vi "LC1_MS_Main.vi"() -> ()   [LabVIEW 2016, in "DNP3_Master_Station_Template.lvlib"]
uses:
  DNP3_Master_Station_Template.lvlib
  Program Files (x86)/National Instruments/LabVIEW 2016/examples/DNP3/Get Started/Master/SubVI/Tab_Master.ctl
  <vilib>/DNP3/DNP3_Master/Response Type.ctl
  <vilib>/Utility/error.llb/DialogType.ctl
  Global_An_In_Var.vi
  Global_An_Out_Mode.vi
  Global_An_Out_Var.vi
  <vilib>/DNP3/DNP3_Master/Send Poll Analog Input By AllPoints (Blocking).vi
  <vilib>/DNP3/DNP3_Master/Read Analog Input.vi
  <vilib>/DNP3/DNP3_Master/Send Analog Output Block (Blocking).vi
  Global_Bin_In_Var.vi
  Global_Bin_Out_Mode.vi
  <vilib>/DNP3/DNP3_Master/Send Poll Binary Input By AllPoints (Blocking).vi
  <vilib>/DNP3/DNP3_Master/Read Binary Input.vi
  <vilib>/DNP3/DNP3_Master/Send CROB (Blocking).vi
  <vilib>/DNP3/DNP3_Master.lvlib
  <resource>/objmgr/dnp3.rc
panel:
  out "object flags":u8[](array[numeric]) format="%08b"
  in  "Channel Setting":T1
  in  "serial port":u16=1
  in  "baud rate (9600)":u32=9600
  in  "Stop":bool
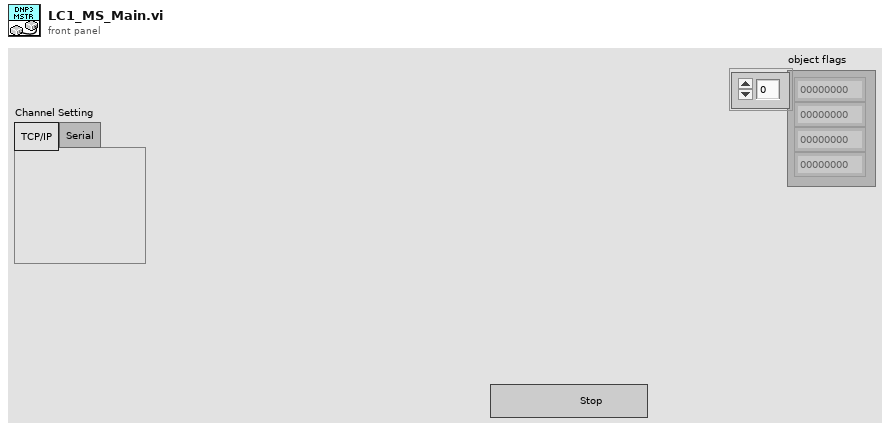
[diagram p1: front panel]
types:
  T1 = typedef "Tab_Master.ctl" = enum32{"TCP/IP", "Serial"}
  T2 = typedef "DNP3_Master.lvlib/Response Type.ctl" = enum16{"Idle", "Buffering", "Pending", "Success", "Failure", "Mismatch", "Status Code", "IIN", "Timeout", "Cancel"}
  T3 = typedef "DialogType.ctl" = u16
  T4 = cluster{"Outstation IP":string, "DNP3 Port":u16, "DNP3 Master Address":u16, "DNP3 Outstation Address":u16}
  T5 = cluster{"DNP3 Master Address":u16, "DNP3 Outstation Address":u16}
  T6 = cluster{bool, "Outstation IP":string, "DNP3 Port":u16, "serial port":u16, "baud rate (9600)":u32}
  T7 = typedef "DNP3_Master.lvlib/Poll Analog Input Variation.ctl" = u8
  T8 = typedef "DNP3_Master.lvlib/Analog Variation.ctl" = u8
  T9 = typedef "DNP3_Master.lvlib/Operation Mode.ctl" = u8
  T10 = typedef "DNP3_Master.lvlib/Analog Info.ctl" = cluster{"index":u16, "value":dbl}
  T11 = typedef "DNP3_Master.lvlib/Poll Binary Input Variation.ctl" = u8
  T12 = typedef "DNP3_Master.lvlib/Crob With Index.ctl" = cluster{"point index":u16, "CROB value":T13}
  T13 = typedef "DNP3_Common.lvlib/crob.ctl" = cluster{"OnTime":u32, "Count":u8, "OffTime":u32, "Control":T14}
  T14 = typedef "DNP3_Common.lvlib/crob_ctrl.ctl" = u8
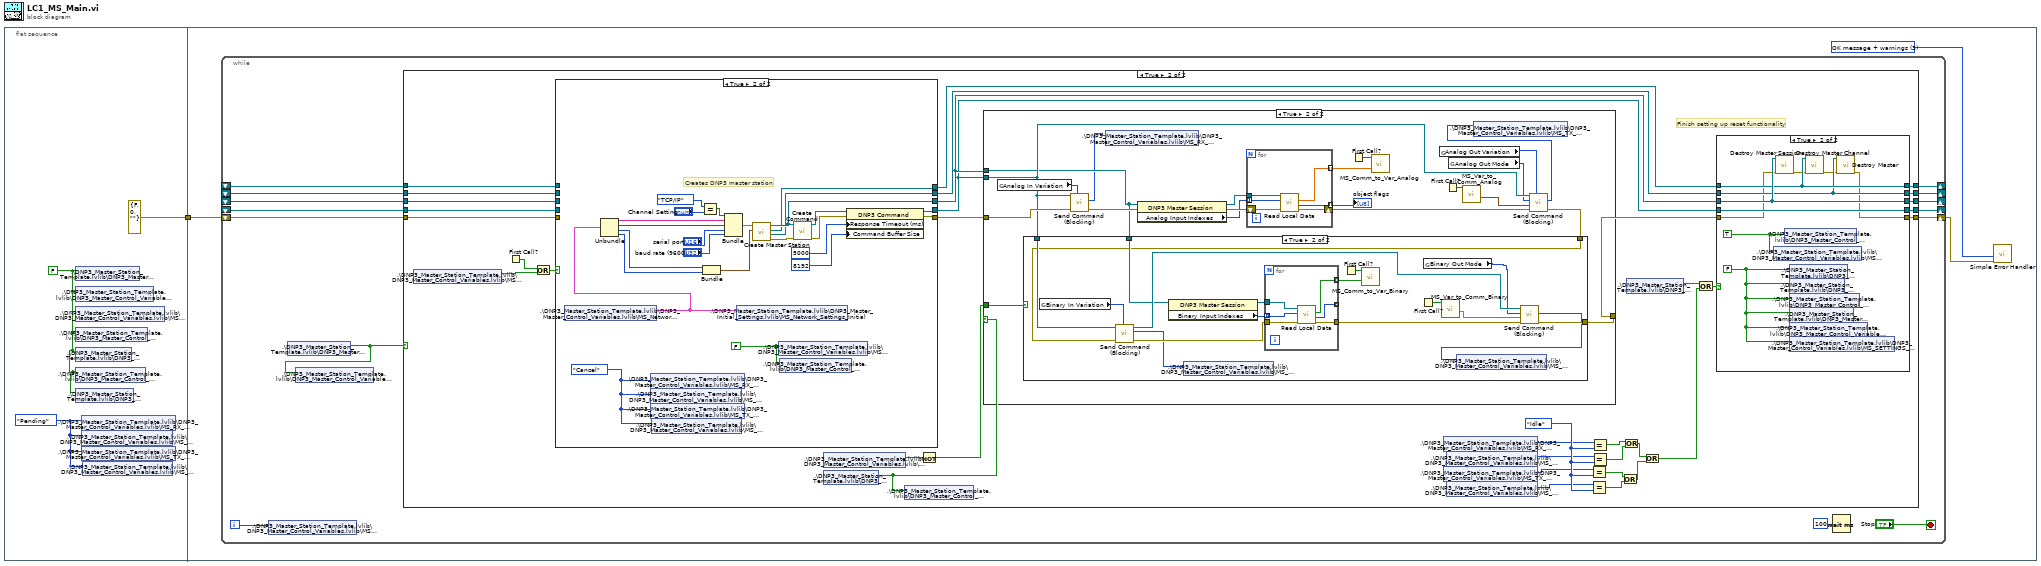
[diagram p0: block diagram]
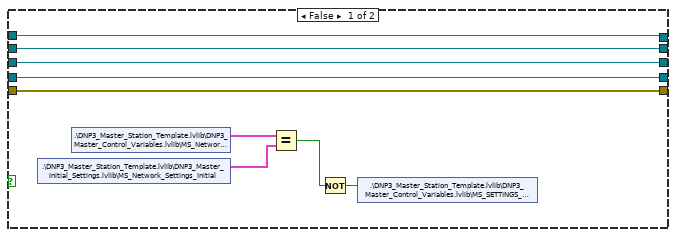
[diagram p4: hidden frame]
diagram:
  n1 = flat-sequence {
    tunnel: [errorcluster {"status"=FALSE, "code"=0, "source"=""} ("error out")] -> w1
    tunnel: w1 -> [w5]
    frame #0 {
      w2 = Response_Type."Pending" ("LC1_MS_RX_Status_Binary")
      w4 = FALSE ("LC1_MS_Enable")
      n2 = shared-variable ".\\DNP3_Master_Station_Template.lvlib\\DNP3_Master_Control_Variables.lvlib\\MS_ENABLE"(w4) -> ()  [unwired: 1 in, 1 out]
      n3 = shared-variable ".\\DNP3_Master_Station_Template.lvlib\\DNP3_Master_Control_Variables.lvlib\\MS_ENABLE_IND"(w4) -> ()  [unwired: 1 in, 1 out]
      n4 = shared-variable ".\\DNP3_Master_Station_Template.lvlib\\DNP3_Master_Control_Variables.lvlib\\MS_RESET_SUCCESS"(w4) -> ()  [unwired: 1 in, 1 out]
      n5 = shared-variable ".\\DNP3_Master_Station_Template.lvlib\\DNP3_Master_Control_Variables.lvlib\\MS_RESET_IND"(w4) -> ()  [unwired: 1 in, 1 out]
      n6 = shared-variable ".\\DNP3_Master_Station_Template.lvlib\\DNP3_Master_Control_Variables.lvlib\\MS_POLL"(w4) -> ()  [unwired: 1 in, 1 out]
      n7 = shared-variable ".\\DNP3_Master_Station_Template.lvlib\\DNP3_Master_Control_Variables.lvlib\\MS_POLL_IND"(w4) -> ()  [unwired: 1 in, 1 out]
      n8 = shared-variable ".\\DNP3_Master_Station_Template.lvlib\\DNP3_Master_Control_Variables.lvlib\\MS_RESET"(w4) -> ()  [unwired: 1 in, 1 out]
      n9 = shared-variable ".\\DNP3_Master_Station_Template.lvlib\\DNP3_Master_Control_Variables.lvlib\\MS_RX_Status_Analog"(w2) -> ()  [unwired: 1 in, 1 out]
      n10 = shared-variable ".\\DNP3_Master_Station_Template.lvlib\\DNP3_Master_Control_Variables.lvlib\\MS_RX_Status_Binary"(w2) -> ()  [unwired: 1 in, 1 out]
      n11 = shared-variable ".\\DNP3_Master_Station_Template.lvlib\\DNP3_Master_Control_Variables.lvlib\\MS_TX_Status_Analog"(w2) -> ()  [unwired: 1 in, 1 out]
      n12 = shared-variable ".\\DNP3_Master_Station_Template.lvlib\\DNP3_Master_Control_Variables.lvlib\\MS_TX_Status_Binary"(w2) -> ()  [unwired: 1 in, 1 out]
    }
    frame #1 {
      w7 = T3 3 items=["no dialog", "OK message", "continue or stop message", "OK message + warnings", "continue/stop + warnings"] ("type of dialog (OK msg:1)")
      n13 = while {
        shift-right: [w18] -> _
        shift-left: _ -> [w21]
        shift-right: [w15] -> _
        shift-left: _ -> [w20]
        shift-right: [w14] -> _
        shift-left: _ -> [w19]
        shift-right: [w16] -> w6
        shift-left: w5 -> [w17]
        shift-right: [w9] -> _
        shift-left: _ -> [w8]
        i -> [w11]
        stop <- "Stop" stop-if-true
        n14 = shared-variable ".\\DNP3_Master_Station_Template.lvlib\\DNP3_Master_Control_Variables.lvlib\\MS_SubVI_Iterations"(w11) -> ()  [unwired: 1 in, 1 out]
        n15 = shared-variable ".\\DNP3_Master_Station_Template.lvlib\\DNP3_Master_Control_Variables.lvlib\\MS_ENABLE"() -> (w10:bool)  [unwired: 1 in, 1 out]
        n16 = shared-variable ".\\DNP3_Master_Station_Template.lvlib\\DNP3_Master_Control_Variables.lvlib\\MS_ENABLE_IND"(w10) -> ()  [unwired: 1 in, 1 out]
        n17 = case shown="True" w10 {
          tunnel: w21 -> [w26 w59]
          tunnel: w20 -> [w25 w58]
          tunnel: w19 -> [w24 w57]
          tunnel: [w26 w55] -> w18
          tunnel: w17 -> [w23 w54]
          tunnel: [w23 w53] -> w16
          tunnel: [w25 w52] -> w15
          tunnel: [w24 w50] -> w14
          tunnel: [w22 w29] -> w9
          tunnel: w8 -> [w22 w27]
          frame False {
          }
          frame True {
            w42 = Response_Type."Idle" ("Analog RX")
            # "Finish setting up reset functionality"
            n18 = shared-variable ".\\DNP3_Master_Station_Template.lvlib\\DNP3_Master_Control_Variables.lvlib\\MS_RESET_SUCCESS"() -> (w35:bool)  [unwired: 1 in, 1 out]
            n19 = First Call?() -> (First Call?: T/F=w61:bool)
            n20 = Or(x=w61, y=w35) -> (x .or. y?=w60:bool)
            n21 = case shown="True" w60 {
              tunnel: [w85 w94] -> w62
              tunnel: [w83 w95] -> w49
              tunnel: [w84 w104] -> w51
              tunnel: w59 -> [w86 _]
              tunnel: w58 -> [w84 _]
              tunnel: w57 -> [w83 _]
              tunnel: [w86 w88] -> w56
              tunnel: w54 -> [w85 _]
              tunnel: [w80 w87] -> w30
              tunnel: w27 -> [w80 _]
              frame False {
                n22 = shared-variable ".\\DNP3_Master_Station_Template.lvlib\\DNP3_Master_Initial_Settings.lvlib\\MS_Network_Settings_Initial"() -> (w81:T4)  [unwired: 1 in, 1 out]
                n23 = shared-variable ".\\DNP3_Master_Station_Template.lvlib\\DNP3_Master_Control_Variables.lvlib\\MS_Network_Settings"() -> (w82:T4)  [unwired: 1 in, 1 out]
                n24 = Equal?(x=w82, y=w81) -> (x = y?=w78:bool)
                n25 = Not(x=w78) -> (.not. x?=w79:bool)
                n26 = shared-variable ".\\DNP3_Master_Station_Template.lvlib\\DNP3_Master_Control_Variables.lvlib\\MS_SETTINGS_CHANGED"(w79) -> ()  [unwired: 1 in, 1 out]
              }
              frame True {
                w89 = Response_Type."Cancel" ("LC1_MS_RX_Status_Binary")
                w97 = FALSE ("MS_Comm_Reset_Ind")
                # "Creates DNP3 master station"
                n27 = shared-variable ".\\DNP3_Master_Station_Template.lvlib\\DNP3_Master_Control_Variables.lvlib\\MS_Network_Settings"() -> (w96:T4)  [unwired: 1 in, 1 out]
                n28 = Unbundle(w96) -> ("Outstation IP"=w103:string, "DNP3 Port"=w102:u16, "DNP3 Master Address"=w101:u16, "DNP3 Outstation Address"=w100:u16)
                n29 = shared-variable ".\\DNP3_Master_Station_Template.lvlib\\DNP3_Master_Control_Variables.lvlib\\MS_RX_Status_Analog"(w89) -> ()  [unwired: 1 in, 1 out]
                n30 = shared-variable ".\\DNP3_Master_Station_Template.lvlib\\DNP3_Master_Control_Variables.lvlib\\MS_RX_Status_Binary"(w89) -> ()  [unwired: 1 in, 1 out]
                n31 = shared-variable ".\\DNP3_Master_Station_Template.lvlib\\DNP3_Master_Control_Variables.lvlib\\MS_TX_Status_Analog"(w89) -> ()  [unwired: 1 in, 1 out]
                n32 = shared-variable ".\\DNP3_Master_Station_Template.lvlib\\DNP3_Master_Control_Variables.lvlib\\MS_TX_Status_Binary"(w89) -> ()  [unwired: 1 in, 1 out]
                n33 = Equal?(x=Tab_Master."TCP/IP" ("Channel Setting"), y="Channel Setting") -> (x = y?=w106:bool)
                n34 = Bundle("DNP3 Master Address"=w101, "DNP3 Outstation Address"=w100) -> (w98:T5)  [unwired: 1 in]
                n35 = Bundle(w106, "Outstation IP"=w103, "DNP3 Port"=w102, "serial port"="serial port", "baud rate (9600)"="baud rate (9600)") -> (w99:T6)  [unwired: 1 in]
                n36 = shared-variable ".\\DNP3_Master_Station_Template.lvlib\\DNP3_Master_Initial_Settings.lvlib\\MS_Network_Settings_Initial"(w96) -> ()  [unwired: 1 in, 1 out]
                n37 = call "Create Master Station.vi"("Session Cluster"=w98, "Channel Cluster"=w99) -> ("error out"=w107:errorcluster, "DNP3 master"=w88:refnum<k21>, "DNP3 channel"=w87:refnum<k21>, "DNP3 master session"=w104:refnum<k21>)  [unwired: 3 in]
                n38 = shared-variable ".\\DNP3_Master_Station_Template.lvlib\\DNP3_Master_Control_Variables.lvlib\\MS_RESET_SUCCESS"(w97) -> ()  [unwired: 1 in, 1 out]
                n39 = shared-variable ".\\DNP3_Master_Station_Template.lvlib\\DNP3_Master_Control_Variables.lvlib\\MS_RESET_IND"(w97) -> ()  [unwired: 1 in, 1 out]
                n40 = call <vilib>:"Create Command.vi"("error in (no error)"=w107, "DNP3 master session"=w104) -> ("error out"=w92:errorcluster, "DNP3 command"=w93:refnum<k21>)  [unwired: 8 in]
                n41 = property class="DNP3 Command"(reference=w93, error in=w92, "Response Timeout (ms)"=u32 5000 ("Misc:Response Timeout (ms)"), "Command Buffer Size"=u32 8192 ("Misc:Command Buffer Size")) -> (reference out=w95:refnum<k21>, error out=w94:errorcluster)
              }
            }
            n42 = shared-variable ".\\DNP3_Master_Station_Template.lvlib\\DNP3_Master_Control_Variables.lvlib\\MS_Disable_Binary"() -> (w44:bool)  [unwired: 1 in, 1 out]
            n43 = shared-variable ".\\DNP3_Master_Station_Template.lvlib\\DNP3_Master_Control_Variables.lvlib\\MS_POLL"() -> (w45:bool)  [unwired: 1 in, 1 out]
            n44 = shared-variable ".\\DNP3_Master_Station_Template.lvlib\\DNP3_Master_Control_Variables.lvlib\\MS_POLL_IND"(w45) -> ()  [unwired: 1 in, 1 out]
            n45 = Not(x=w44) -> (.not. x?=w43:bool)
            n46 = case shown="True" w45 {
              tunnel: w49 -> [_ w125]
              tunnel: w51 -> [_ w124]
              tunnel: w62 -> [w111 w128]
              tunnel: [w111 w122] -> w48
              tunnel: w43 -> [_ w121]
              frame False {
              }
              frame True {
                n47 = global read "Global_An_In_Var.vi" "Analog In Variation"() -> (w114:T7)
                n48 = call-poly <vilib>:"Send Command (Blocking).vi"("variation (Default)"=w114, "error in (no error)"=w128, "DNP3 command in"=w125) -> ("error out"=w131:errorcluster, "response status"=w120:T2)  [unwired: 6 in, 1 out]
                n49 = shared-variable ".\\DNP3_Master_Station_Template.lvlib\\DNP3_Master_Control_Variables.lvlib\\MS_RX_Status_Analog"(w120) -> ()  [unwired: 1 in, 1 out]
                n50 = property class="DNP3 Master Session"(reference=w124, error in=w131) -> (reference out=w129:refnum<k21>, error out=w130:errorcluster, "Analog Input Indexes"=w127:u16[])
                n51 = for {
                  tunnel: [w160] -> w117 mode=indexing
                  tunnel: [w159] -> w132 mode=indexing
                  tunnel: w129 -> [w158]
                  tunnel: w127 -> [w157] mode=indexing
                  shift-right: [w161] -> w126
                  shift-left: w130 -> [w162]
                  n52 = call-poly <vilib>:"Read Local Data.vi"("error in (no error)"=w162, "point index"=w157, "DNP3 master session in"=w158) -> ("error out"=w161:errorcluster, "object flags"=w159:u8, "value"=w160:dbl)  [unwired: 5 in, 1 out]
                }
                "object flags" <- w132
                n53 = First Call?() -> (First Call?: T/F=w116:bool)
                n54 = call "MS_Comm_to_Var_Analog.vi"("Array"=w117, "Boolean"=w116) -> ()  [unwired: 10 in]
                n55 = global read "Global_An_Out_Var.vi" "Analog Out Variation"() -> (w112:T8)
                n56 = First Call?() -> (First Call?: T/F=w115:bool)
                n57 = global read "Global_An_Out_Mode.vi" "Analog Out Mode"() -> (w113:T9)
                n58 = call "MS_Var_to_Comm_Analog.vi"("Boolean"=w115) -> ("values"=w118:T10[])  [unwired: 10 in]
                n59 = call-poly <vilib>:"Send Command (Blocking).vi"("variation"=w112, "error in (no error)"=w126, "values"=w118, "mode"=w113, "DNP3 command in"=w125) -> ("error out"=w123:errorcluster, "response status"=w119:T2)  [unwired: 4 in, 1 out]
                n60 = case shown="True" w121 {
                  tunnel: w125 -> [_ w145]
                  tunnel: w124 -> [_ w144]
                  tunnel: w123 -> [w133 w143]
                  tunnel: [w133 w142] -> w122
                  frame False {
                  }
                  frame True {
                    n61 = global read "Global_Bin_In_Var.vi" "Binary In Variation"() -> (w135:T11)
                    n62 = call-poly <vilib>:"Send Command (Blocking).vi"("variation (Default)"=w135, "error in (no error)"=w143, "DNP3 command in"=w145) -> ("error out"=w146:errorcluster, "response status"=w141:T2, "DNP3 command out"=w147:refnum<k21>)  [unwired: 6 in]
                    n63 = property class="DNP3 Master Session"(reference=w144) -> (reference out=w149:refnum<k21>, "Binary Input Indexes"=w148:u16[])  [unwired: 1 in, 1 out]
                    n64 = shared-variable ".\\DNP3_Master_Station_Template.lvlib\\DNP3_Master_Control_Variables.lvlib\\MS_RX_Status_Binary"(w141) -> ()  [unwired: 1 in, 1 out]
                    n65 = for {
                      tunnel: [w156] -> w150
                      tunnel: [w155] -> _ mode=indexing
                      tunnel: [w154] -> w138 mode=indexing
                      tunnel: w149 -> [w153]
                      tunnel: w148 -> [w152] mode=indexing
                      tunnel: w146 -> [w151]
                      n66 = call-poly <vilib>:"Read Local Data.vi"("error in (no error)"=w151, "point index"=w152, "DNP3 master session in"=w153) -> ("error out"=w156:errorcluster, "object flags"=w155:u8, "value"=w154:bool)  [unwired: 5 in, 1 out]
                    }
                    n67 = First Call?() -> (First Call?: T/F=w137:bool)
                    n68 = call "MS_Comm_to_Var_Binary.vi"("Input Data"=w138, "Boolean"=w137) -> ()  [unwired: 10 in]
                    n69 = First Call?() -> (First Call?: T/F=w136:bool)
                    n70 = global read "Global_Bin_Out_Mode.vi" "Binary Out Mode"() -> (w134:T9)
                    n71 = call "MS_Var_to_Comm_Binary.vi"("Boolean"=w136) -> ("Array"=w139:T12[])  [unwired: 10 in]
                    n72 = call-poly <vilib>:"Send Command (Blocking).vi"("error in (no error)"=w150, "CROB values"=w139, "mode"=w134, "DNP3 command in"=w147) -> ("error out"=w142:errorcluster, "response status"=w140:T2)  [unwired: 5 in, 1 out]
                    n73 = shared-variable ".\\DNP3_Master_Station_Template.lvlib\\DNP3_Master_Control_Variables.lvlib\\MS_TX_Status_Binary"(w140) -> ()  [unwired: 1 in, 1 out]
                  }
                }
                n74 = shared-variable ".\\DNP3_Master_Station_Template.lvlib\\DNP3_Master_Control_Variables.lvlib\\MS_TX_Status_Analog"(w119) -> ()  [unwired: 1 in, 1 out]
              }
            }
            n75 = shared-variable ".\\DNP3_Master_Station_Template.lvlib\\DNP3_Master_Control_Variables.lvlib\\MS_RX_Status_Analog"() -> (w34:T2)  [unwired: 1 in, 1 out]
            n76 = shared-variable ".\\DNP3_Master_Station_Template.lvlib\\DNP3_Master_Control_Variables.lvlib\\MS_TX_Status_Analog"() -> (w32:T2)  [unwired: 1 in, 1 out]
            n77 = shared-variable ".\\DNP3_Master_Station_Template.lvlib\\DNP3_Master_Control_Variables.lvlib\\MS_RX_Status_Binary"() -> (w33:T2)  [unwired: 1 in, 1 out]
            n78 = shared-variable ".\\DNP3_Master_Station_Template.lvlib\\DNP3_Master_Control_Variables.lvlib\\MS_TX_Status_Binary"() -> (w31:T2)  [unwired: 1 in, 1 out]
            n79 = Equal?(x=w32, y=w42) -> (x = y?=w37:bool)
            n80 = Equal?(x=w31, y=w42) -> (x = y?=w38:bool)
            n81 = Equal?(x=w34, y=w42) -> (x = y?=w39:bool)
            n82 = Equal?(x=w33, y=w42) -> (x = y?=w36:bool)
            n83 = Or(x=w37, y=w38) -> (x .or. y?=w40:bool)
            n84 = Or(x=w39, y=w36) -> (x .or. y?=w41:bool)
            n85 = shared-variable ".\\DNP3_Master_Station_Template.lvlib\\DNP3_Master_Control_Variables.lvlib\\MS_RESET"() -> (w46:bool)  [unwired: 1 in, 1 out]
            n86 = Or(x=w41, y=w40) -> (x .or. y?=w28:bool)
            n87 = Or(x=w46, y=w28) -> (x .or. y?=w47:bool)
            n88 = case shown="True" w47 {
              tunnel: w56 -> [w67 w72]
              tunnel: [w67 w72] -> w55
              tunnel: w48 -> [w66 w71]
              tunnel: [w66 w68] -> w53
              tunnel: [w65 w74] -> w52
              tunnel: w51 -> [w65 w74]
              tunnel: [w64 w77] -> w50
              tunnel: w49 -> [w64 w77]
              tunnel: w30 -> [w63 w73]
              tunnel: [w63 w73] -> w29
              frame False {
              }
              frame True {
                w75 = FALSE ("MS_Comm_Reset")
                w76 = TRUE ("MS_Comm_Reset_Succesful")
                n89 = shared-variable ".\\DNP3_Master_Station_Template.lvlib\\DNP3_Master_Control_Variables.lvlib\\MS_RESET_SUCCESS"(w76) -> ()  [unwired: 1 in, 1 out]
                n90 = call <vilib>:"Destroy Master Session.vi"("error in (no error)"=w71, "DNP3 master session in"=w74) -> ("error out"=w70:errorcluster)  [unwired: 8 in, 1 out]
                n91 = shared-variable ".\\DNP3_Master_Station_Template.lvlib\\DNP3_Master_Control_Variables.lvlib\\MS_RESET_IND"(w76) -> ()  [unwired: 1 in, 1 out]
                n92 = shared-variable ".\\DNP3_Master_Station_Template.lvlib\\DNP3_Master_Control_Variables.lvlib\\MS_RESET"(w75) -> ()  [unwired: 1 in, 1 out]
                n93 = shared-variable ".\\DNP3_Master_Station_Template.lvlib\\DNP3_Master_Control_Variables.lvlib\\MS_POLL"(w75) -> ()  [unwired: 1 in, 1 out]
                n94 = shared-variable ".\\DNP3_Master_Station_Template.lvlib\\DNP3_Master_Control_Variables.lvlib\\MS_POLL_IND"(w75) -> ()  [unwired: 1 in, 1 out]
                n95 = shared-variable ".\\DNP3_Master_Station_Template.lvlib\\DNP3_Master_Control_Variables.lvlib\\MS_ENABLE"(w75) -> ()  [unwired: 1 in, 1 out]
                n96 = shared-variable ".\\DNP3_Master_Station_Template.lvlib\\DNP3_Master_Control_Variables.lvlib\\MS_ENABLE_IND"(w75) -> ()  [unwired: 1 in, 1 out]
                n97 = shared-variable ".\\DNP3_Master_Station_Template.lvlib\\DNP3_Master_Control_Variables.lvlib\\MS_SETTINGS_CHANGED"(w75) -> ()  [unwired: 1 in, 1 out]
                n98 = call <vilib>:"Destroy Master Channel.vi"("error in (no error)"=w70, "DNP3 channel in"=w73) -> ("error out"=w69:errorcluster)  [unwired: 8 in, 1 out]
                n99 = call <vilib>:"Destroy Master.vi"("error in (no error)"=w69, "DNP3 master"=w72) -> ("error out"=w68:errorcluster)  [unwired: 9 in]
              }
            }
          }
        }
        n100 = Wait (ms)(milliseconds to wait=u32 100) -> ()  [unwired: 1 out]
      }
      n101 = call <vilib>:"Simple Error Handler.vi"("type of dialog (OK msg:1)"=w7, "error in (no error)"=w6) -> ()  [unwired: 3 in, 5 out]
    }
  }
